vi "Initialize Truck.vi"(6 "Interior cargo capacity":dbl, 8 "model":string, 9 "make":string, 10 "Bed cargo capacity":dbl, 11 "truck in":refnum<class "Truck.lvclass">) -> (3 "truck out":refnum<class "Truck.lvclass">)   [LabVIEW 2011, in "Truck.lvclass"]
doc: "This method initializes the data members of the class \"Truck.\""
uses:
  Truck.lvclass
  Truck.lvclass/Truck.ctl
  Vehicle/Vehicle.lvclass
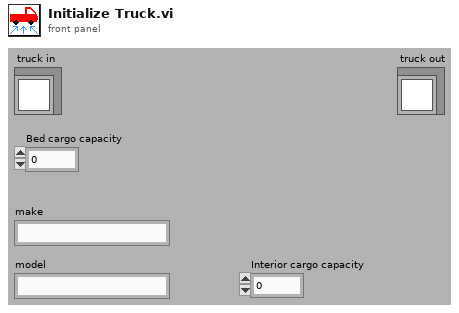
[diagram p1: front panel]
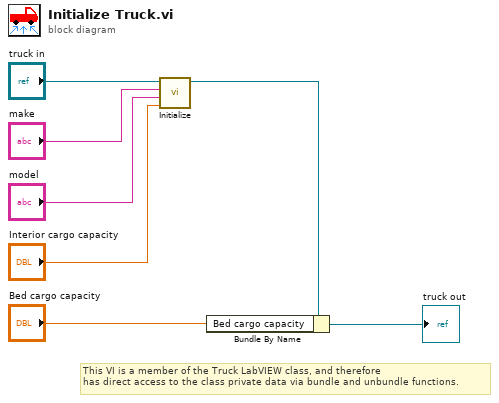
[diagram p0: block diagram]
diagram:
  # "This VI is a member of the Truck LabVIEW class, and therefore\nhas direct access to the class private data via bundle and unbundle functions."
  n1 = call "Initialize.vi"("Interior cargo capacity"="Interior cargo capacity", "model"="model", "make"="make", "vehicle in"="truck in") -> ("vehicle out"=w4:refnum<class "Truck.lvclass">)  [unwired: 7 in]
  n2 = Bundle By Name(cluster=w4, "Bed cargo capacity"="Bed cargo capacity") -> (→"truck out":refnum<class "Truck.lvclass">)
